vi "check_password.vi"(1 "Ref":T1) -> (0 "result？":bool)   [LabVIEW 2015]
uses:
  <vilib>/registry/registry.llb/Registry RtKey.ctl
  <vilib>/registry/registry.llb/Read Registry Value Simple STR.vi
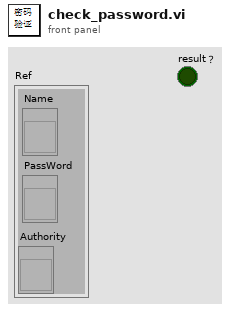
[diagram p1: front panel]
types:
  T1 = cluster{"Name":refnum<vi>, "PassWord":refnum<vi>, "Authority":refnum<vi>}
  T2 = typedef "Registry RtKey.ctl" = enum32{"HKEY_CLASSES_ROOT", "HKEY_CURRENT_USER", "HKEY_LOCAL_MACHINE", "HKEY_USERS", "HKEY_PERFORMANCE_DATA", "HKEY_CURRENT_CONFIG", "HKEY_DYN_DATA"}
  T3 = typedef "Registry refnum.ctl" = refnum<k1>
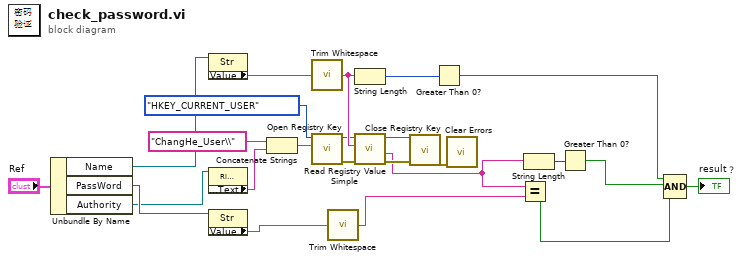
[diagram p0: block diagram]
diagram:
  n1 = Unbundle By Name("Ref") -> ("Name"=w9:refnum<vi>, "PassWord"=w8:refnum<vi>, "Authority"=w7:refnum<vi>)
  n2 = property class="Str"(reference=w9) -> ("Value"=w11:string)  [unwired: 1 in, 2 out]
  n3 = property class="Ring (严格)"(reference=w7) -> ("RingText.Text"=w18:string)  [unwired: 1 in, 2 out]
  n4 = property class="Str"(reference=w8) -> ("Value"=w12:string)  [unwired: 1 in, 2 out]
  n5 = Concatenate Strings("ChangHe_User\\" ("字符串"), w18) -> (w20:string)
  n6 = call <vilib>:"Trim Whitespace.vi"("string"=w11) -> ("trimmed string"=w23:string)  [unwired: 1 in]
  n7 = call <vilib>:"Open Registry Key.vi"("subkey"=w20, "root key (HKEY_LOCAL_MACHINE)"=Registry_RtKey."HKEY_CURRENT_USER") -> ("error out"=w21:errorcluster, "refnum out"=w22:T3)  [unwired: 8 in]
  n8 = call <vilib>:"Trim Whitespace.vi"("string"=w12) -> ("trimmed string"=w2:string)  [unwired: 1 in]
  n9 = String Length(string=w23) -> (length=w13:i32)
  n10 = call-poly <vilib>:"Read Registry Value Simple.vi"("error in (no error)"=w21, "value"=w23, "refnum"=w22) -> ("error out"=w5:errorcluster, "String/Binary data"=w1:string, "refnum out"=w6:T3)  [unwired: 3 in, 1 out]
  n11 = call <vilib>:"Close Registry Key.vi"("error in (no error)"=w5, "refnum"=w6) -> ("error out"=w4:errorcluster)  [unwired: 5 in]
  n12 = Greater Than 0?(x=w13) -> (x > 0?=w15:bool)
  n13 = call <vilib>:"Clear Errors.vi"("error in (no error)"=w4) -> ()  [unwired: 5 in, 2 out]
  n14 = Equal?(x=w1, y=w2) -> (x = y?=w24:bool)
  n15 = String Length(string=w1) -> (length=w14:i32)
  n16 = Greater Than 0?(x=w14) -> (x > 0?=w16:bool)
  n17 = Compound Arithmetic op=AND ("复合运算")(w15, w16, w24) -> (→"result？":bool)
